vi "Meas_ADJ_Status.vi"(6 "NumRows":u32, 8 "에러 입력(에러 없음)":errorcluster, 11 "Measured_ADJ in":refnum<vi>[](array[refnum])) -> (0 "에러 출력":errorcluster, 3 "Measured_ADJ out":refnum<vi>[](array[refnum]))   [LabVIEW 2020]
uses:
  Variables/Global_Cal Info.vi
  Variables/Global_Constant.vi
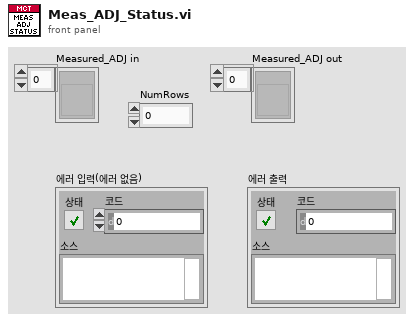
[diagram p1: front panel]
types:
  T1 = typedef "Clst_Cal Info Global.ctl" = cluster{"등록번호":string, "의뢰기관":string, "기기명":string, "제작회사":string, "형식":string, "기기번호":string, "소분류코드":string, "세부분류코드":string, "교정주기":string, "접수번호":string, "교정일자":string, "교정절차서 1":string, "교정절차서 2":string, "교정절차서 3":string, "접수확인자":string, "인증교정자":string, "기술책임자":string, "KOLAS 유무":string, "진행상태":string, "의뢰기관코드":string, "입고형태":string, "영문성적서?":bool, "합불판정?":bool, "부록?":bool, "절차서번호 1":string, "절차서번호 2":string, "절차서번호 3":string, "교정방식":string, "부서명":string}
  T2 = enum8{"Enabled", "Disabled", "Disabled and Grayed Out"}
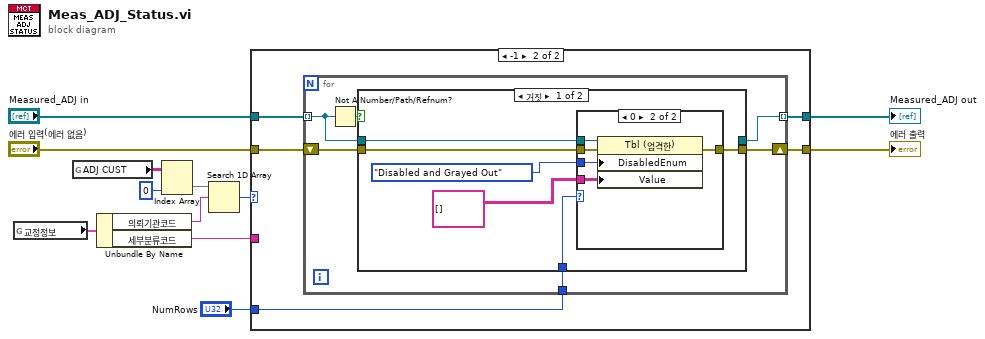
[diagram p0: block diagram]
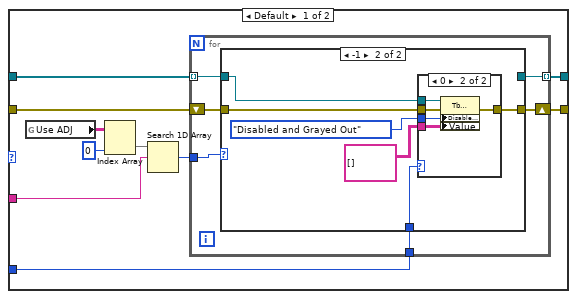
[diagram p2: hidden frame]
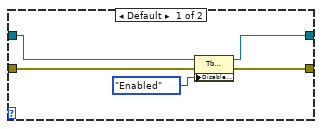
[diagram p3: hidden frame]
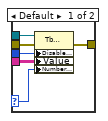
[diagram p4: hidden frame]
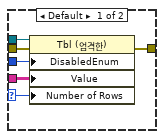
[diagram p5: hidden frame]
diagram:
  n1 = global read "Global_Cal Info.vi" "교정정보"() -> (w9:T1)
  n2 = global read "Global_Constant.vi" "ADJ CUST"() -> (w7:string[][])
  n3 = Unbundle By Name(w9) -> ("의뢰기관코드"=w4:string, "세부분류코드"=w8:string)
  n4 = Index Array(array=w7, index (col)=0 ("비활성화된 인덱스 (열)")) -> (element=w5:string[])  [unwired: 1 in]
  n5 = Search 1D Array(1D array=w5, element=w4) -> (index of element=w3:i32)  [unwired: 1 in]
  n6 = case shown="-1" w3 {
    tunnel: "Measured_ADJ in" -> [w22 w55]
    tunnel: [w21 w54] -> w11
    tunnel: "에러 입력(에러 없음)" -> [w20 w53]
    tunnel: w8 -> [w16 _]
    tunnel: [w14 w52] -> w2
    tunnel: "NumRows" -> [w13 w51]
    frame Default {
      n7 = global read "Global_Constant.vi" "Use ADJ"() -> (w19:string[][])
      n8 = Index Array(array=w19, index (col)=0 ("비활성화된 인덱스 (열)")) -> (element=w17:string[])  [unwired: 1 in]
      n9 = Search 1D Array(1D array=w17, element=w16) -> (index of element=w15:i32)  [unwired: 1 in]
      n10 = for {
        shift-right: [w24] -> w21
        shift-left: w20 -> [w26]
        tunnel: w22 -> [w27] mode=indexing
        tunnel: w15 -> [w28]
        tunnel: [w25] -> w14 mode=indexing
        tunnel: w13 -> [w23]
        n11 = case shown="-1" w28 {
          tunnel: w27 -> [w33 w39]
          tunnel: w26 -> [w32 w38]
          tunnel: [w31 _] -> w25
          tunnel: [w29 w36] -> w24
          tunnel: w23 -> [_ w35]
          frame Default {
            n12 = property class="Tbl (엄격한)"(reference=w33, error in=w32, "DisabledEnum"=T2."Enabled" ("비활성화")) -> (reference out=w31:refnum<vi>, error out=w29:errorcluster)
          }
          frame -1 {
            n13 = case shown="0" w35 {
              selector: w35 -> [w41 _]
              tunnel: w39 -> [w45 w50]
              tunnel: w38 -> [w44 w49]
              tunnel: T2."Disabled and Grayed Out" ("비활성화") -> [w43 w48]
              tunnel: [w42 w47] -> w36
              tunnel: string[][] [] -> [w40 w46]
              frame Default {
                n14 = property class="Tbl (엄격한)"(reference=w45, error in=w44, "DisabledEnum"=w43, "Value"=w40, "Number of Rows"=w41) -> (error out=w42:errorcluster)  [unwired: 1 out]
              }
              frame 0 {
                n15 = property class="Tbl (엄격한)"(reference=w50, error in=w49, "DisabledEnum"=w48, "Value"=w46) -> (error out=w47:errorcluster)  [unwired: 1 out]
              }
            }
          }
        }
      }
    }
    frame -1 {
      n16 = for {
        shift-right: [w60] -> w54
        shift-left: w53 -> [w61]
        tunnel: w55 -> [w59] mode=indexing
        tunnel: [w57] -> w52 mode=indexing
        tunnel: w51 -> [w56]
        n17 = Not A Number/Path/Refnum?(number/path/refnum=w59) -> (NaN/Path/Refnum?=w58:bool)
        n18 = case shown="거짓" w58 {
          tunnel: w61 -> [w67 w80]
          tunnel: [w66 w80] -> w60
          tunnel: w59 -> [w65 w79]
          tunnel: [_ w79] -> w57
          tunnel: w56 -> [w63 _]
          frame False {
            n19 = case shown="0" w63 {
              selector: w63 -> [w69 _]
              tunnel: w67 -> [w73 w78]
              tunnel: [w72 w77] -> w66
              tunnel: w65 -> [w71 w76]
              tunnel: T2."Disabled and Grayed Out" ("비활성화") -> [w70 w75]
              tunnel: string[][] [] -> [w68 w74]
              frame Default {
                n20 = property class="Tbl (엄격한)"(reference=w71, error in=w73, "DisabledEnum"=w70, "Value"=w68, "Number of Rows"=w69) -> (error out=w72:errorcluster)  [unwired: 1 out]
              }
              frame 0 {
                n21 = property class="Tbl (엄격한)"(reference=w76, error in=w78, "DisabledEnum"=w75, "Value"=w74) -> (error out=w77:errorcluster)  [unwired: 1 out]
              }
            }
          }
          frame True {
          }
        }
      }
    }
  }
  "에러 출력" <- w11
  "Measured_ADJ out" <- w2
